vi "observacao.vi"() -> ()   [LabVIEW 2018, in "Shared_160.lvlib"]
uses:
  Shared_160.lvlib
  Control 1.ctl
  System.Windows.Forms
  Global_Telescopio.vi
panel:
  out "statusReadTime":u32
  in  "Internal Dew Point":dbl
  in  "Dew Point 2":dbl
  in  "Humidity 2":dbl
  in  "Wind Speed 2":dbl
  in  "LEAF 2":i32
  in  "ExternalTracking":bool caption="non-sideral"
  out "externalNST":bool
  in  "VARIABLE \nTRACKING":bool
  out "LED VAR TRACKING":bool
  out "LED GUIDER":bool
  out "Led Chave Dome":bool
  out "LED MOUNT":bool
  in  "GUIDER":bool
  in  "DOME":bool
  in  "MOUNT":bool
  out "Weather rec. time":timestamp
  in  "Default":string="DEFAULT"
  out "angCup":string caption="DOME Pos"
  out "TargetCup":string caption="DOME Tar"
  out "domeRisc":bool
  out "element":string
  out "size(s)":i32
  out "timeStatShutterAlert":i32
  out "sendCommandShutter":bool
  out "shutterTimeOld":i32
  out "LEAF":i32
  out "Flag ativo DEC":bool
  out "Flag ativo AH":bool
  out "Flag de erro p/ apagar lampada":bool
  in  "erro lig":i32=3
  in  "erro des":i32=3
  in  "xxz":string
  out "Flag desligar":bool
  out "Flag ligar":bool
  out "Flag Stop":bool
  in  "AUX LAMPADA":bool
  out "Apontou":bool caption="Working Area"
  in  "AUX ABA":bool
  in  "error in (no error)":errorcluster
  out "AH_Destino":dbl format="%.9g"
  out "CONT DEC UTILS":i32
  out "CR DEC UTILS":i32
  out "CONT AH UTILS":i32
  out "CR AH UTILS":i32
  out "Erro PROTEC":i32=5
  out "Erro Lim":i32=5
  out "Flag Alarm":bool
  out "alarm Time":timestamp
  in  "LedPointing":bool=TRUE
  in  "Case Ct":bool=TRUE
  in  "Case Constant\n(See Context Help) 12":bool=TRUE
  in  "Case Constant\n(See Context Help) 11":bool
  in  "Case Constant\n(See Context Help) 8":bool=TRUE
  in  "Case Constant\n(See Context Help) 7":bool=TRUE
  in  "Case Constant\n(See Context Help) 6":bool
  in  "Case Constant\n(See Context Help) 5":bool
  in  "TRUE=HORA\nFALSE=GRAU":bool=TRUE
  in  "Case Constant\n(See Context Help) 4":bool
  in  "Case Constant\n(See Context Help) 3":bool
  in  "Case Constant\n(See Context Help) 2":bool
  in  "Case Constant\n(See Context Help)":bool
  out "TA3":u32
  out "TA2":u32
  out "TF2":u32
  out "TF1":u32
  out "TA1":u32
  out "Tick Cupula":u32
  out "T2 3":u32
  in  "ESTADO ABRIR":string
  in  "ESTADO FECHAR":string
  out "T2 2":u32
  out "T1 2":u32
  out "T2":u32
  out "T1":u32
  out "DEC":string="00 00 00,00"
  out "Hour Angle 2":string="00 00 0,00" caption="AH"
  in  "TIMER TICK":u32
  in  "STOP":bool
  in  "News":bool
  out "AtmosferaStr":string
  in  "BtShutterClose":bool caption="DOME SHUTTER"
  out "HA obs":dbl
  out "Time to Limit":string
  in  "Clear All Messages":bool
  out "FiltroDuplo":bool
  out "ObjCentrado":bool
  out "Timeout PROT":u32
  out "LIMITE":bool
  in  "DestCUP":i16
  in  "DestAH":dbl
  in  "DestDEC":dbl
  in  "M_CUP":i32
  out "TimeoutCUP 2":u32
  out "TimeoutAH 2":u32
  out "TimeoutDEC 2":u32
  out "error out":errorcluster
  out "TUBO_STAT":string
  out "CUP_STAT":string
  out "DEC_STAT":string
  out "AH_STAT":string
  out "FOCO_ENC":string
  out "DEC_ENC":string
  out "AH_ENC":string
  out "RA on Target":bool
  in  "BtOnTatget":bool
  out "Offset DEC":dbl format="%#.2f"
  out "Offset RA":dbl format="%#.2f"
  out "Mount Fine Movement":bool
  out "Mount Gross Movement":bool
  out "subarray":string[][](array[string])
  in  "sair":bool
  out "Saida Path string":string
  out "AUX EDITA RA":string caption="Name"
  out "Sideral time":string caption="ST"
  out "UT":string
  out "FLAG SET COORD":bool
  out "AUX EDITA PMDEC":string caption="Name"
  out "AUX EDITA PMRA":string caption="Name"
  out "AUX EDITA EPOCH":string caption="Name"
  out "AUX EDITA DEC":string caption="Name"
  out "AUX EDITA Name":string caption="Name"
  out "Hour Angle":string="00 00 0,00"
  in  "DECTARGET":string
  in  "AHTARGET":string
  out "Zenital angle":dbl
  out "SlideEnviromental":dbl(slide) caption="Progress ..." scale=0.0..100.0
  out "RA AUX":string
  out "EPOCH AUX":string
  out "SYSTEM MESSAGES":string
  out "Data Acquisition Activity":bool
  out "Auto guider Activity":bool
  out "Security Zone":bool
  out "Precess Data out-of-date":bool
  out "Weather data received":bool
  out "Plataform":bool
  out "B...":bool
  out "Shutter opened":bool
  out "DEC on Target":bool
  out "Dome on Target":bool
  out "Remote User in Control":bool
  out "Air Mass":dbl
  out "Epoch":dbl
  out "Right Ascention":string="00 00 00,00"
  out "Declination":string="00 00 00,00"
  out "Azimuth":dbl
  out "Wind Chill":dbl
  out "Boolean 11":bool
  out "Wind Dir":string
  in  "Int/Ext":bool=TRUE
  out "Temperature":dbl
  out "Humidity":dbl
  out "Dew Point":dbl
  out "Wind Speed":dbl
  out "Pressure":dbl
  out "NAME":string
  out "DEC":string
  out "RA":string
  in  "Tab Control":T1(tab)=enum."Test Only"
  in  "PictureBox":refnum<k24>(container)
  out "pressão atm":string
  out "hum local":string
  out "Temp amb":string
  out "C. AH":i32
  out "DOMO_ENC":string
  out "Proteção":bool
  in  "M_PROT":i32
  out "dt":u32
  out "TUBO":bool[](array[boolean])
  out "CUP":bool[](array[boolean])
  out "DEC":bool[](array[boolean])
  out "RA":bool[](array[boolean])
  in  "statCUP":i32
  in  "statAH":i32
  in  "statDEC":i32
  out "statCUP 2":i32
  out "TimeoutCUP":u32
  out "Azimute cup":u16
  out "PosCUP":i16
  out "dtAUX2":u32
  out "dtAUX3":u32
  out "PosAH":dbl
  out "PosDEC":dbl
  out "dec=":bool
  out "ah=":bool
  in  "CR AH":i32
  in  "CR DEC":i32
  out "C. DEC":i32
  in  "M_AH":i32
  in  "M_DEC":i32
  out "cmdT":string
  in  "Stop All":bool
  in  "Setup, Pointing & Guiding":T2(tab)=enum."POINTING"
  in  "RA Max 2":i32 min=-6 max=23
  in  "RA Min 2":i32 min=-6 max=23
  out "Erro":bool
  in  "MAG Max":dbl min=-9.0 max=100.0
  in  "MAG Min":dbl min=-9.0 max=25.0
  in  "DEC Max":i32 min=-90 max=90
  in  "DEC Min":i32 min=-90 max=90
  in  "RA Max":i32 caption="AH Max" min=-6 max=23
  in  "RA Min":i32 caption="AH Min" min=-6 max=23
  in  "Filter RA":bool
  in  "Slide old":i32
  out "Tot Linhas":i32
  in  "Open BSC":bool
  in  "Slide":dbl(slide) min=0.0 max=24.0 step=0.024 scale format="%#_3g"
  in  "EDIT":bool
  in  "Insert":bool
  out "List File":string
  in  "Upload":bool
  in  "Open":bool
  in  "Save AS":bool
  in  "Save":bool
  in  "Clear ALL":bool
  in  "SET coord":bool
  in  "Delete":bool
  in  "Multicolumn Listbox":i32[](listbox)
  out "ScaleMin":string
  out "ScaleMax":string
  out "DEC obs":dbl format="%.9f"
  out "RA obs":dbl format="%.9f"
  in  "ChkPointPrecessed":bool
  in  "Processa Centragem":bool
  out "PM_DEC":string
  out "PM_RA":string
  out "LedPointing":bool caption="Telescope Pointing"
  out "TimeoutAH":u32
  out "TimeoutDEC":u32
  out "AtualDEC":dbl format="%.9f"
  out "MeanDEC":string
  out "MeanRA":string
  in  "MAG":string
  out "Zenital Angle":string
  out "Air Mass":string
  out "Tempo Obs":string
  in  "BtPointPrecess":bool
  in  "ChkCalGlobal":bool=TRUE
  in  "ChkCalLocal":bool caption="Use Local Zero"
  in  "ChkPoinLampOFF":bool=TRUE
  in  "ChkPointRNA":bool
  in  "ChkModel":bool=TRUE
  in  "ChkWindDown":bool
  in  "ChkOpenShutter":bool
  in  "ChkDomeEnable":bool
  out "LedPointWorkArea":bool caption="Working Area"
  in  "BtTargetPoint":bool
  out "StrPointTargetDEC":string caption="Declination"
  out "StrPointTargetRA":string caption="Right Ascension"
  in  "BtPointObjClear":bool
  in  "StrPointObjPMDEC":string caption="DEC Proper Motion"
  in  "StrPointObjPMRA":string caption="RA Proper Motion"
  in  "StrPointObjName":string caption="Name"
  in  "StrPointObjEpoch":string caption="Epoch"
  in  "StrPointObjDEC":string caption="Declination"
  in  "StrPointObjRA":string caption="Right Ascension"
  out "MOV_IDX_DEC":bool
  out "MOV_IDX_AH":bool
  out "LatchDeslocDEC":dbl caption="DEC"
  out "LatchDeslocRA":dbl caption="RA"
  in  "ClearDeslocDEC":bool
  in  "ClearDeslocRA":bool
  out "DeslocDEC":dbl caption="DEC" format="%#.1f"
  out "DeslocRA":dbl caption="RA" format="%#.1f"
  in  "Delete Calagem":bool
  in  "Global":bool caption="Local"
  in  "Calagem":bool
  in  "Up HS":bool
  in  "Right HS":bool
  in  "Down HS":bool
  in  "Left HS":bool
  in  "Velocity (arcsec/sec)":i32(slide) min=0 max=600 scale=0.0..600.0
  in  "BtPrecGO":bool
  in  "BtPrecCentrar":bool
  in  "PreciseOffsetDEC":dbl caption="DEC" min=-10000.0 max=10000.0 step=1.0 format="%.3g"
  in  "PreciseOffsetRA":dbl caption="RA . cos(delta)" min=-10000.0 max=10000.0 step=1.0 format="%.3g"
  in  "Habilita Movimento":bool=TRUE
  in  "Y STAR":i32=1 min=1 max=400 step=1
  in  "X STAR":i32=1 min=1 max=400 step=1
  in  "XY CENTER":bool
  in  "Y CENTER":i32=1 min=1 max=400 step=1
  in  "X CENTER":i32=1 min=1 max=400 step=1
  in  "ClearRA":bool
  in  "ClearDEC":bool
  in  "DEC RATE":i32 min=-2000 max=2000 step=1
  in  "RA  RATE":i32 min=-2000 max=2000 step=1
  in  "focusStop":bool
  in  "Velocity":dbl(slide)=1.0 caption="(max = 500 u/s)" min=0.1 max=100.0 step=1.0 scale=0.1..100.0
  in  "focusHome":bool
  out "focusStatus":string="            Focus Status"
  out "focuAlarm":bool caption="Motor temp."
  out "focusHoming":bool caption="Homing"
  out "focusMoving":bool caption="Moving"
  out "focusConnected":bool
  out "focusInitialized":bool
  in  "SetDefaultFocus":bool
  out "Foco":dbl(slide) caption="1" scale=0.0..50000.0
  in  "Setpoint":dbl=200.0 caption="Target" min=0.0 max=50700.0 step=1.0
  in  "focusGo":bool
  in  "Focus +":bool caption="Focus Out (+)"
  in  "Focus -":bool caption="Focus In (-)"
  in  "New Angle":string="    0.0"
  out "Default Angle":string="      0.00"
  in  "SetRotatorDefAngle":bool
  in  "Set Rotator Angle":bool
  out "Rotator Angle":string="  0.00" caption="for  GUIDING"
  in  "OpenShutterPassword":string caption="Senha para Abrir"
  in  "BtShutterClose":bool
  in  "BtShutterOpen":bool
  out "trapeiraAberta":bool caption="Open"
  out "trapeiraMovendo":bool caption="Moving"
  out "trapeiraFechada":bool caption="Closed"
  out "Command":string
  in  "CCW":bool
  in  "BtParavStop":bool
  in  "BtParavUp":bool
  in  "BtParavDown":bool
  out "StatDome":string caption="Control State"
  in  "BtDomeSTOP":bool
  in  "BtDomeGO":bool caption="DOME"
  in  "DomeNewPos":i32=30 caption="New Position" min=1 max=360
  out "AngCup":i16 caption="Position"
  in  "CW":bool
  in  "BtUtilPark":bool
  out "LED ACTION":bool
  out "LED MODE":bool
  in  "ACTION":bool
  in  "MODE":bool
  in  "PROTEÇÃO":bool
  in  "STOP":bool
  in  "Enable Centragem":bool=TRUE
  in  "GO":bool
  in  "StrPointObjDEC 2":string caption="DEC"
  in  "StrPointObjRA 2":string caption="AH"
  out "MOVING":bool
  in  "FLAT-FIELD":bool
  in  "ECASS":bool
  in  "BtUtilZenith":bool
  in  "TabInstrumento":T3(tab)=enum."Cam 1"
  out "Posição Rede":i32=10 caption="Largura da Fenda" min=10 max=5000 step=1
  in  "HomePrisma":T4 caption="DOME"
  in  "HomeEspelho":T4 caption="DOME"
  in  "HomeFenda":T4 caption="DOME"
  in  "IronArc":bool=TRUE
  out "Boolean":bool
  out "Largura da Fenda 2":dbl=10.0 caption="Largura da Fenda" min=10.0 max=5000.0 step=1.0
  in  "Prisma das Lâmpadas":bool
  out "Position":string
  in  "Largura da Fenda":dbl=10.0 min=10.0 max=5000.0 step=1.0
  in  "Go Largura da Fenda":bool caption="DOME"
  in  "Angulo da rede de difração":i32=10 caption="Ângulo da Rede" min=10 max=99989 step=1
  in  "Go Angulo de Difração":bool caption="DOME"
  in  "Incand":bool=TRUE
  in  "Neon":bool=TRUE
  in  "Cathode":bool=TRUE
  out "Ang. Fenda":dbl
  in  "Go_Coudé":bool
  in  "Radio Buttons":enum32{"Azul", "Visível", "Vermelho"}(radio)
  out "EndTime":u32
  out "ledAzul":bool
  out "ledVisivel":bool
  out "ledVermelho":bool
  in  "MENSAGEM":string="EM MOVIMENTO"
  out "MENSAGEM 2":string="EM MOVIMENTO"
  out "#2":bool
  out "#3":bool
  out "#4":bool
  out "PosSecundario":bool
  out "Cjto_3":bool
  out "EspAtual":string
  out "parou":bool
  out "parou 2":bool
  out "Posição Espelho":dbl=10.0 caption="Largura da Fenda" min=10.0 max=5000.0 step=1.0
  out "parou 3":bool
  out "Output Message":string
  in  "stopEcass":bool
  out "SlideEcass":u8(slide) caption="Espelho movendo..." max=100 scale=0.0..100.0
  out "LedRep":bool
  out "LedCal":bool
  in  "Sent_EspLampCass":bool
  out "LedHe":bool
  out "LedNe":bool
  in  "He-Ar":bool
  in  "Ne":bool
  in  "Mensage Alarme":string="To light up close the Shutter !"
  out "CoudeSel":bool
  in  "Coude":bool
  in  "BtCalFlatField":bool
  in  "ChkCalLamp4":bool
  in  "ChkCalLamp3":bool
  in  "ChkCalLamp2":bool
  in  "ChkCalLamp1":bool
  in  "BtCalTurnOff":bool
  in  "BtCalTurnOn":bool
  out "StrongSel":bool
  out "MediumSel":bool
  out "WeakSel":bool
  in  "Strong":bool
  in  "Medium":bool
  in  "Weak":bool
  # "TELESCOPE CONTROL SYSTEM\nPICO DOS DIAS OBSERVATORY"
  # "Status Information"
  # "System Positions"
  # "Environmental Status"
  # "(+/-2)"
  # "mBar"
  # "INT"
  # "EXT"
  # "o"
  # "C"
  # "Km/h"
  # "%"
  # "o"
  # "C"
  # "o"
  # "C"
  # "CLOUSURE LIMITS"
  # "Wind Speed            >  70 Km/h\nRelative Humidity    >  97 %\nInternal Dewpoint  <  0.5  C\nExternal Dewpoint <  1.0  C"
  # "OBJECT"
  # "TRACKING ENABLE"
  # "Conector 4"
  # "Conector 3"
  # "ALARME\nATENÇÃO\nERROS\nOCUPADO"
  # "Proteção\n\nTracking\nVar_Track"
  # "PLATAF\nLCB\nTRAP\nPARAV"
  # "Rapido\nLigeiro\nFino\nRun"
  # "Rapido\nCW\nCCW\nMoving"
  # "Motor\nIDX_Rdy\nManual"
  # "TRAP_RUN\nTRAP_FCH\nTRAP_ABT"
  # "BSC FILTERS"
  # "LIST FILE"
  # "OBJECT INPUT"
  # "TARGET"
  # "OPTIONS"
  # "MANUAL OFFSET"
  # "PRECISE OFFSET"
  # "N"
  # "E"
  # "W"
  # "arcsec"
  # "arcsec"
  # "S"
  # "DISPLACEMENT"
  # "CALAGEM"
  # "PODE NÃO FUNCIONAR CORRETAMENTE!"
  # "STAR CENTERING"
  # "AUTO-GUIDER COORDINATES"
  # "INTERNAL VAR. TRACKING"
  # "1) Entrar X e Y do cursor do Autoguider correspondente à posição de centragem nas entradas X CENTER e Y CENTER. \n2) Após apontamento, entrar em X STAR e Y STAR os valores de X e Y do Autoguider com o \"Guide Box\" sobre o objeto apontado. \n3) Clicar em MOVE STAR TO CENTER."
  # "(instrument)"
  # "May take many\ntens of seconds"
  # "Continuous Movement"
  # "%"
  # "ATENÇÃO:\nO Rotator ainda não está integrado ao sistema de controle e como sua posição afeta a guiagem, sempre que o rotator for girado manualmente é necessário digitar o valor de sua nova posição no controle \"New Angle\" e pressionar \"SET NEW\".\n\nPressionar \"SET NEW\" ou \"SET DEFAULT\" não gira o rotator!"
  # "ROTATION"
  # "WINDSCREEN"
  # "SHUTTER"
  # "Covers"
  # "FIXED POSITIONS"
  # "Acquisition System\nON TARGET command"
  # "Select one Mirrror"
  # "Mirror #2"
  # "Mirror #3"
  # "Mirrors Drivers"
  # "Lâmpadas de Calibração"
  # "Espelho das Lâmpadas de Calibração"
  # "Posição"
  # "Repouso"
  # "Ativo"
  # "LIGA"
  # "LIGA"
  # "DESL."
  # "DESL."
  # "Espelho do Eucalyptus"
  # "Roda de filtros"
  # "Posição"
  # "Repouso"
  # "Ativo"
  # "Espelho de Campo"
  # "Recuar"
  # "Avançar"
  # "Rápido"
  # "Lento"
  # "CALIBRATION LAMPS"
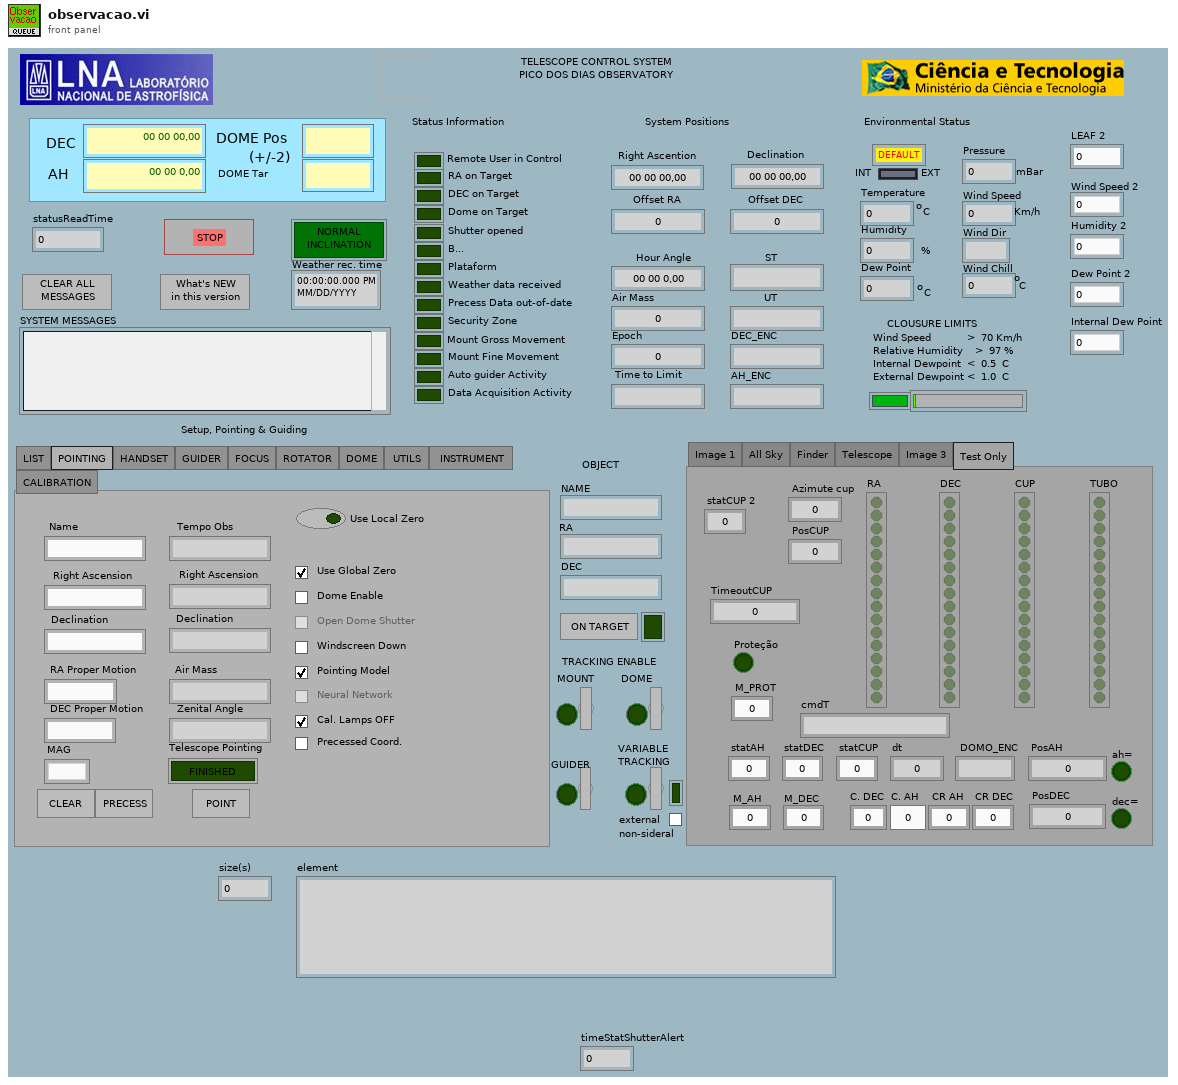
[diagram p1: front panel]
types:
  T1 = enum32{"Image 1", "All Sky", "Finder", "Telescope", "Image 3", "Test Only"}
  T2 = enum32{"LIST", "POINTING", "HANDSET", "GUIDER", "FOCUS", "ROTATOR", "DOME", "UTILS ", " INSTRUMENT ", "CALIBRATION"}
  T3 = enum32{"Coude", "Casseg.", "Eucalyp.", "Cam 1", "Cam 2", "Cam IV.", "Polarim.", "Fotrap"}
  T4 = typedef "Control 1.ctl" = bool
  T5 = enum8{"Enabled", "Disabled", "Disabled and Grayed Out"}
  T6 = enum32{"Page Enabled", "Page Disabled", "Page Disabled & Grayed"}
  T7 = enum16{"open", "replace", "create", "open or create", "replace or create", "replace or create with confirmation"}
  T8 = enum16{"open", "open or create", "create or replace", "create"}
  T9 = enum16{"open", "open or create", "create or replace", "create", "open (read only)"}
  T10 = typedef "LVRemotePanelConnectionsTypeDef.ctl" = cluster{"VI Name":string, "Remote":string, "UserName":string, "Port":i32, "Status":enum32{"Viewing", "Waiting For Control", "Controlling"}, "Create Time":timestamp, "Status Time":timestamp, "Control End Time":timestamp}[]
  T11 = cluster{"absolute":bool, "alarm":bool, "broker":string, "cmd":cluster{"clientId":dbl, "clientTransactionId":dbl, "clientName":string, "action":string}, "connected":bool, "controller":string, "device":string, "error":string, "homing":bool, "initialized":bool, "isMoving":bool, "maxSpeed":dbl, "maxStep":dbl, "position":dbl, "tempComp":bool, "tempCompAvailable":bool, "temperature":dbl, "timestamp":string, "version":string}
  T12 = cluster{"clientId":dbl, "clientTransactionId":dbl, "clientName":string, "action":string}
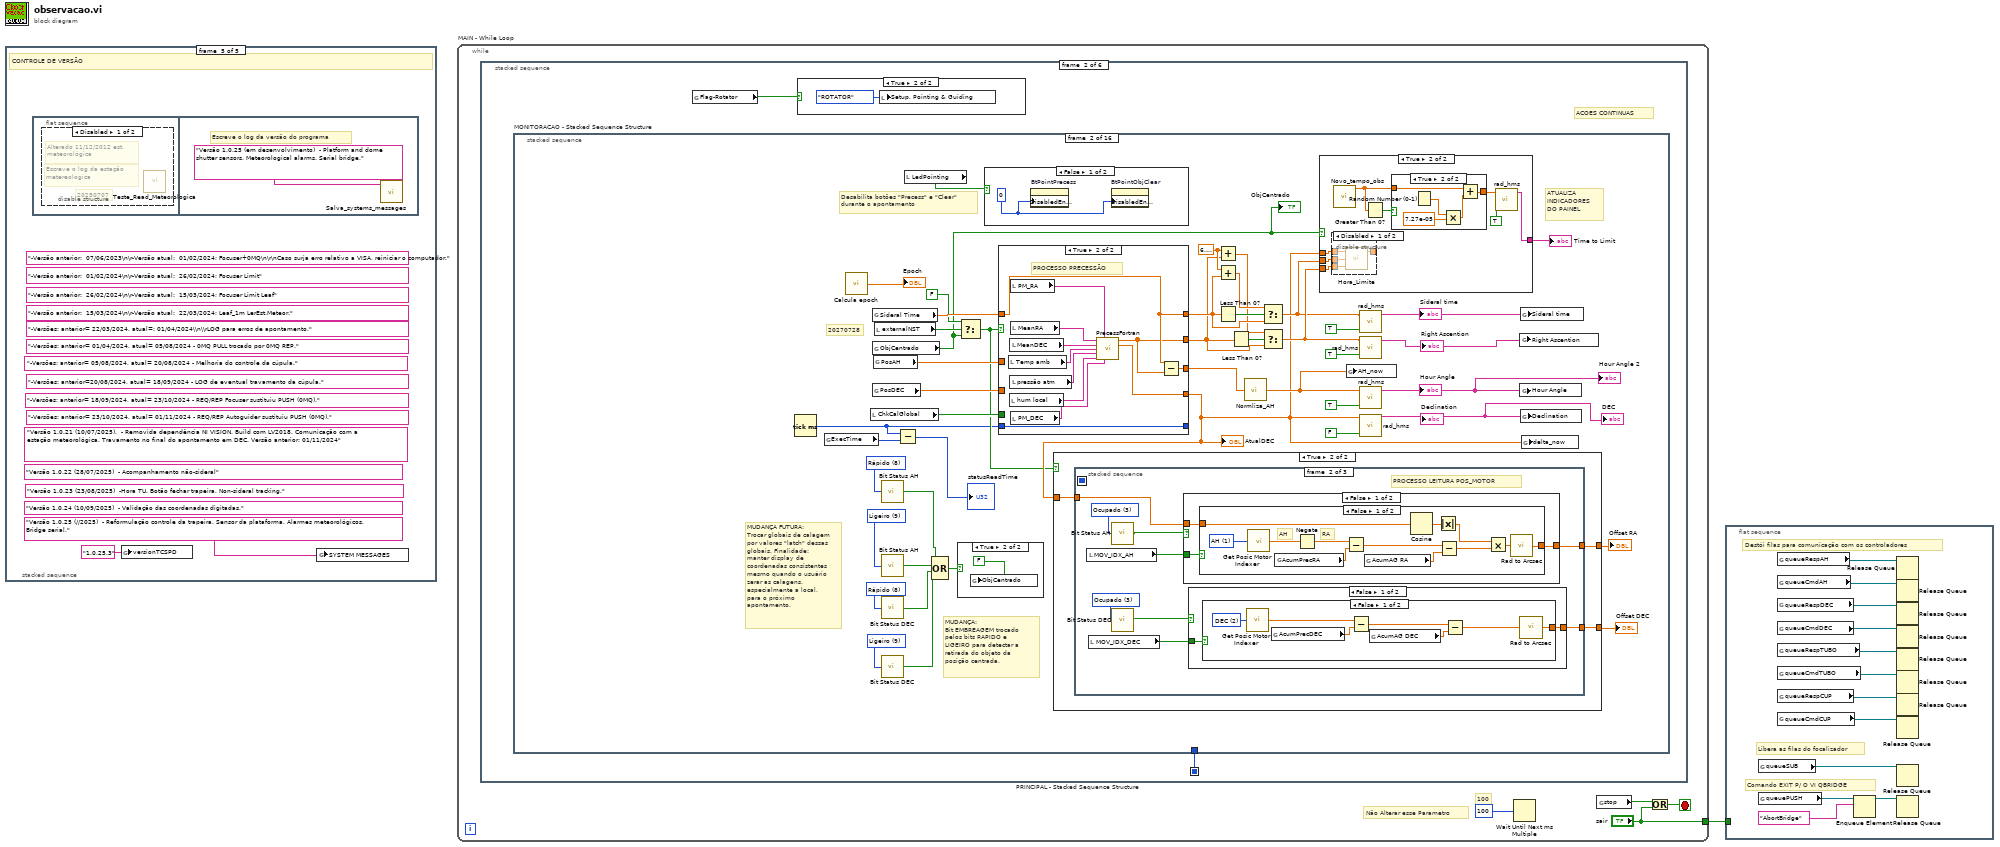
[diagram p0: block diagram]
diagram:
  n1 = stacked-sequence {
    frame #0 {
      w3 = ""
      w5 = 0 ("estado")
      w4 = ""
      w6 = TRUE ("ChkDomeEnable")
      w2 = FALSE ("Set aux")
      # "RESET DE VARIÁVEIS E CONTROLES"
      n2 = local write "FLAG SET COORD"(w2) -> ()
      n3 = local write "DEC on Target"(w2) -> ()
      n4 = local write "Dome on Target"(w2) -> ()
      n5 = local write "MOUNT"(w2) -> ()
      n6 = local write "ACTION"(w2) -> ()
      n7 = local write "GO"(w2) -> ()
      n8 = local write "MOV_IDX_AH"(w2) -> ()
      n9 = local write "MOV_IDX_DEC"(w2) -> ()
      n10 = local write "Flag ativo AH"(w2) -> ()
      n11 = local write "MOVING"(w2) -> ()
      n12 = local write "Flag ativo DEC"(w2) -> ()
      n13 = local write "RA on Target"(w2) -> ()
      n14 = local write "Erro"(w2) -> ()
      n15 = local write "ChkPointPrecessed"(w2) -> ()
      n16 = local write "ChkOpenShutter"(w2) -> ()
      n17 = local write "Enable Centragem"(w2) -> ()
      n18 = local write "Cathode"(w2) -> ()
      n19 = local write "Neon"(w2) -> ()
      n20 = local write "Incand"(w2) -> ()
      n21 = local write "Apontou"(w2) -> ()
      n22 = local write "Precess Data out-of-date"(w2) -> ()
      n23 = local write "Flag Stop"(w2) -> ()
      n24 = local write "MODE"(w2) -> ()
      n25 = local write "LED ACTION"(w2) -> ()
      n26 = local write "LED MODE"(w2) -> ()
      n27 = local write "Flag de erro p/ apagar lampada"(w2) -> ()
      n28 = local write "ExternalTracking"(w2) -> ()
      n29 = local write "externalNST"(w2) -> ()
      n30 = local write "trapeiraFechada"(w2) -> ()
      n31 = local write "trapeiraMovendo"(w2) -> ()
      n32 = local write "trapeiraAberta"(w2) -> ()
      n33 = global write "Global_Telescopio.vi" "Default Met"(w2) -> ()
      n34 = global write "Global_Telescopio.vi" "Flag-Rotator"(w2) -> ()
      n35 = global write "Global_Telescopio.vi" "Centragem Via Aquisicao"(w2) -> ()
      n36 = global write "Global_Telescopio.vi" "Botão GO = STOP"(w2) -> ()
      n37 = global write "Global_Telescopio.vi" "AQ Offset Mov"(w2) -> ()
      n38 = global write "Global_Telescopio.vi" "STOP ALL"(w2) -> ()
      n39 = global write "Global_Telescopio.vi" "Bit RX Aquis"(w2) -> ()
      n40 = global write "Global_Telescopio.vi" "Bit RX Guider"(w2) -> ()
      n41 = global write "Global_Telescopio.vi" "Correção Guider"(w2) -> ()
      n42 = global write "Global_Telescopio.vi" "CalGlobal"(w2) -> ()
      n43 = global write "Global_Telescopio.vi" "CalLocal"(w2) -> ()
      n44 = global write "Global_Telescopio.vi" "ObjCentrado"(w2) -> ()
      n45 = global write "Global_Telescopio.vi" "LIMITE"(w2) -> ()
      n46 = global write "Global_Telescopio.vi" "ExtDEC correction"(w2) -> ()
      n47 = global write "Global_Telescopio.vi" "ExtRA correction"(w2) -> ()
      n48 = global write "Global_Telescopio.vi" "ExtDEC_shift"(w3) -> ()
      n49 = global write "Global_Telescopio.vi" "ExtRA_shift"(w3) -> ()
      n50 = local write "TIMER TICK"(w5) -> ()
      n51 = local write "erro lig"(w5) -> ()
      n52 = local write "erro des"(w5) -> ()
      n53 = local write "statDEC"(w5) -> ()
      n54 = local write "statAH"(w5) -> ()
      n55 = local write "statCUP"(w5) -> ()
      n56 = local write "Tick Cupula"(w5) -> ()
      n57 = local write "CR AH"(w5) -> ()
      n58 = local write "CR DEC"(w5) -> ()
      n59 = global write "Global_Telescopio.vi" "CupStartPos"(w5) -> ()
      n60 = local write "StrPointTargetRA"(w4) -> ()
      n61 = local write "StrPointTargetDEC"(w4) -> ()
      n62 = local write "AUX EDITA RA"(w4) -> ()
      n63 = local write "AUX EDITA EPOCH"(w4) -> ()
      n64 = local write "AUX EDITA PMRA"(w4) -> ()
      n65 = local write "Tempo Obs"(w4) -> ()
      n66 = local write "RA"(w4) -> ()
      n67 = local write "DEC"(w4) -> ()
      n68 = local write "NAME"(w4) -> ()
      n69 = local write "MAG"(w4) -> ()
      n70 = local write "StrPointObjName"(w4) -> ()
      n71 = local write "StrPointObjRA"(w4) -> ()
      n72 = local write "StrPointObjDEC"(w4) -> ()
      n73 = local write "StrPointObjEpoch"(w4) -> ()
      n74 = local write "StrPointObjPMRA"(w4) -> ()
      n75 = local write "StrPointObjPMDEC"(w4) -> ()
      n76 = local write "AUX EDITA Name"(w4) -> ()
      n77 = local write "AUX EDITA DEC"(w4) -> ()
      n78 = local write "AUX EDITA PMDEC"(w4) -> ()
      n79 = local write "ScaleMin"(w4) -> ()
      n80 = local write "Zenital Angle"(w4) -> ()
      n81 = local write "Air Mass"(w4) -> ()
      n82 = local write "Position"(w4) -> ()
      n83 = local write "angCup"(w4) -> ()
      n84 = local write "Position"(w4) -> ()
      n85 = local write "angCup"(w4) -> ()
      n86 = local write "ScaleMax"(w4) -> ()
      n87 = local write "ChkDomeEnable"(w6) -> ()
      n88 = local write "AUX ABA"(w6) -> ()
      n89 = local write "AUX LAMPADA"(w6) -> ()
    }
    frame #1 {
      w8 = "C:\\TCS\\SETUP\\METEOR_DEFAULT.DAT"
      w11 = TRUE ("GUIDING")
      w14 = string[][] [] ("Item Names")
      w16 = T5."Enabled" ("Disabled")
      # "TU safe"
      # "INICIALIZAÇÃO DE PROPRIEDADES"
      n90 = property on="Setup, Pointing & Guiding" class="TabCtl (strict)"() -> ("Pages"=w13:refnum<vi>[])  [unwired: 2 in, 2 out]
      n91 = for {
        tunnel: w13 -> [w32] mode=indexing
        # "HABILITA TODAS AS ABAS"
        n92 = property class="Page"(reference=w32, "Page Enabled State"=T6."Page Enabled") -> ()  [unwired: 1 in, 2 out]
      }
      n93 = property on="Setup, Pointing & Guiding" class="TabCtl (strict)"("Page Selector Visible"=TRUE) -> ()  [unwired: 2 in, 2 out]
      n94 = property on="BtPointObjClear" class="Bool"("DisabledEnum"=w16) -> ()  [unwired: 2 in, 2 out]
      n95 = property on="BtPointPrecess" class="Bool"("DisabledEnum"=w16) -> ()  [unwired: 2 in, 2 out]
      n96 = property on="PROTEÇÃO" class="Bool (strict)"("Disabled"=w16) -> ()  [unwired: 2 in, 2 out]
      n97 = property on="FLAT-FIELD" class="Bool (strict)"("Disabled"=w16) -> ()  [unwired: 2 in, 2 out]
      n98 = property on="BtUtilZenith" class="Bool (strict)"("Disabled"=w16) -> ()  [unwired: 2 in, 2 out]
      n99 = property on="ECASS" class="Bool (strict)"("Disabled"=w16) -> ()  [unwired: 2 in, 2 out]
      n100 = property on="BtUtilPark" class="Bool (strict)"("Disabled"=w16) -> ()  [unwired: 2 in, 2 out]
      n101 = property on="ACTION" class="Bool (strict)"("Disabled"=T5."Disabled and Grayed Out") -> ()  [unwired: 2 in, 2 out]
      n102 = property on="Setup, Pointing & Guiding" class="TabCtl (strict)"("MultColors"=TRUE ("Allow Multiple Colors")) -> ()  [unwired: 2 in, 2 out]
      n103 = property on="LedPointWorkArea" class="Bool (strict)"("Visible"=TRUE ("GUIDING")) -> ()  [unwired: 2 in, 2 out]
      n104 = property on="Mensage Alarme" class="Str"("Visible"=FALSE, "Blinking"=TRUE) -> ()  [unwired: 2 in, 2 out]
      n105 = property on="LedPointing" class="Bool (strict)"("Visible"=FALSE ("Set aux")) -> ()  [unwired: 2 in, 2 out]
      n106 = String To Path(string=w8) -> (path=w10:path)
      n107 = call <vilib>:"Check if File or Folder Exists.vi"("path"=w10) -> ("file or folder exists?"=w9:bool)  [unwired: 8 in, 2 out]
      n108 = case shown="False" w9 {
        tunnel: w8 -> [w27 _]
        frame False {
          n109 = global read "Global_Telescopio.vi" "weatherCfgDef"() -> (w30:string[])
          n110 = Build Array(w30) -> (w29:string[][])
          n111 = Transpose 2D Array(2D array=w29) -> (transposed array=w28:string[][])
          n112 = call "salvaexel.vi"("appended array"=w28, "file name p/ exell"=w27) -> ()  [unwired: 1 in, 1 out]
        }
        frame True {
        }
      }
      n113 = call "Get host time.vi"() -> ("BR current time"=w7:timestamp)  [unwired: 8 in, 3 out]
      n114 = control-ref of="BtTargetPoint"() -> (w19:refnum<vi>)
      n115 = control-ref of="Erro"() -> (w21:refnum<vi>)
      n116 = property on="domeRisc" class="Bool"("Visible"=FALSE ("Set aux")) -> ()  [unwired: 2 in, 2 out]
      n117 = property on="domeRisc" class="Bool"("Blinking"=w11) -> ()  [unwired: 2 in, 2 out]
      n118 = global write "Global_Telescopio.vi" "weather160 PUB time"(w7) -> ()
      n119 = global write "Global_Telescopio.vi" "weather 0MQ last time"(w7) -> ()
      n120 = property class="Bool (strict)"(reference=w21, "Boolean Text.Text"="") -> ()  [unwired: 1 in, 2 out]
      n121 = property class="Bool"(reference=w19, "Boolean Text.Text"="POINT") -> ()  [unwired: 1 in, 2 out]
      n122 = property on="Multicolumn Listbox" class="MCListbox (strict)"("Item Names"=w14) -> ()  [unwired: 2 in, 2 out]
      n123 = local write "subarray"(w14) -> ()
      "domeRisc" <- w11
    }
    frame #2 {
      w35 = "REPOUSO" ("y")
      # "20250927 Cria filas para comunicação com Bridge serial.vi"
      # "TU safe"
      # "MUDANÇA 22/6/11:\nÂngulo do rotator muda ao reiniciar o PC."
      # "Iinicializando o timer do shutter"
      # "INICIALIZAÇÃO DE CONTROLES E FILAS DE COMUNICAÇÃO"
      n124 = stacked-sequence {
        frame #0 {
          n125 = Obtain Queue(name (unnamed)="queueCmdAH", element data type="") -> (queue out=w48:refnum<queue>)  [unwired: 3 in, 2 out]
          n126 = global write "Global_Telescopio.vi" "queueCmdAH"(w48) -> ()
          n127 = Obtain Queue(name (unnamed)="queueRespAH", element data type="") -> (queue out=w45:refnum<queue>)  [unwired: 3 in, 2 out]
          n128 = global write "Global_Telescopio.vi" "queueRespAH"(w45) -> ()
        }
        frame #1 {
          n129 = Obtain Queue(name (unnamed)="queueCmdDEC", element data type="") -> (queue out=w54:refnum<queue>)  [unwired: 3 in, 2 out]
          n130 = global write "Global_Telescopio.vi" "queueCmdDEC"(w54) -> ()
          n131 = Obtain Queue(name (unnamed)="queueRespDEC", element data type="") -> (queue out=w51:refnum<queue>)  [unwired: 3 in, 2 out]
          n132 = global write "Global_Telescopio.vi" "queueRespDEC"(w51) -> ()
        }
        frame #2 {
          n133 = Obtain Queue(name (unnamed)="queueCmdTUBO", element data type="") -> (queue out=w60:refnum<queue>)  [unwired: 3 in, 2 out]
          n134 = global write "Global_Telescopio.vi" "queueCmdTUBO"(w60) -> ()
          n135 = Obtain Queue(name (unnamed)="queueRespTUBO", element data type="") -> (queue out=w57:refnum<queue>)  [unwired: 3 in, 2 out]
          n136 = global write "Global_Telescopio.vi" "queueRespTUBO"(w57) -> ()
        }
        frame #3 {
          n137 = Obtain Queue(name (unnamed)="queueCmdCUP", element data type="") -> (queue out=w66:refnum<queue>)  [unwired: 3 in, 2 out]
          n138 = global write "Global_Telescopio.vi" "queueCmdCUP"(w66) -> ()
          n139 = Obtain Queue(name (unnamed)="queueRespCUP", element data type="") -> (queue out=w63:refnum<queue>)  [unwired: 3 in, 2 out]
          n140 = global write "Global_Telescopio.vi" "queueRespCUP"(w63) -> ()
        }
      }
      n141 = call "Get host time.vi"() -> ("BR current time"=→"alarm Time":timestamp)  [unwired: 8 in, 3 out]
      n142 = global read "Global_Telescopio.vi" "rotator_def"() -> (w34:string)
      n143 = global read "Global_Telescopio.vi" "Instrum"() -> (w39:u16)
      n144 = local write "Multicolumn Listbox"(i32[] [0] ("Multicolumn Listbox")) -> ()
      n145 = local write "ESTADO FECHAR"(w35) -> ()
      n146 = local write "TabInstrumento"(w39) -> ()
      n147 = property on="TabInstrumento" class="TabCtl (strict)"("Disabled"=u8 0) -> ()  [unwired: 2 in, 2 out]
      n148 = local write "ESTADO ABRIR"(w35) -> ()
      n149 = local write "Rotator Angle"(w34) -> ()
      n150 = local write "Default Angle"(w34) -> ()
      n151 = global write "Global_Telescopio.vi" "guide_ang"(w34) -> ()
      n152 = local write "StatDome"("Stopped" ("Status")) -> ()
      n153 = local write "xxz"("inicio") -> ()
      "Flag Alarm" <- FALSE ("Visible")
      "shutterTimeOld" <- 0 ("shutterTimeOld")
      "sendCommandShutter" <- FALSE ("writeShutterLog")
      "timeStatShutterAlert" <- 0 ("timeStatShutterAlert")
    }
    frame #3 {
      w69 = u8 0 ("Disabled")
      w70 = "OFF"
      w74 = "focusQueue" ("string")
      w75 = ""
      w84 = u16 4 items=["ZERO", "AH", "DEC", "TUBO", "CUP"] ("Controlador")
      w83 = u16 3 items=["ZERO", "AH", "DEC", "TUBO", "CUP"] ("Controlador")
      w81 = u16 2 items=["ZERO", "AH", "DEC", "TUBO", "CUP"] ("Controlador")
      w85 = "PROG" ("Comando")
      w86 = "RESET" ("Comando")
      w80 = u16 1 items=["ZERO", "AH", "DEC", "TUBO", "CUP"] ("Controlador")
      # "Inicializa ClientTransactionId"
      # "Cria as filas de comunicação\ncom 0MQ_Bridge_Foco.vi"
      # "ZeroMQ"
      # "0- Alarme\n1-Atenção\n2-Erro\n3-Ocupado\n******************\n4-Proteção\n5-Embreagem\n6-Tracking\n7-Var.Track\n8-Rápido\n9-Ligeiro\n10-Médio\n11-Lento\n12-Em movimento\n13-TBD\n14-TBF\n15-TBF\n16-TBF"
      # "RESET DOS CONTROLADORES E INICIALIZAÇÃO DAS FILAS DO FOCALIZADOR"
      n154 = call "Monta Comando.vi"("Comando"=w86, "Dispositivo"=w85, "Controlador"=w80) -> ()  [unwired: 2 in, 5 out]
      n155 = property on="Focus +" class="Bool (strict)"("BoolText.Text"=w70) -> ()  [unwired: 2 in, 2 out]
      n156 = property on="Focus -" class="Bool (strict)"("BoolText.Text"=w70) -> ()  [unwired: 2 in, 2 out]
      n157 = Concatenate Strings(w74, "PUSH" ("string")) -> (w77:string)
      n158 = Concatenate Strings(w74, "SUB" ("string")) -> (w76:string)
      n159 = call "Monta Comando.vi"("Comando"=w86, "Dispositivo"=w85, "Controlador"=w81) -> ()  [unwired: 2 in, 5 out]
      n160 = Wait (ms)(milliseconds to wait=u32 2000) -> ()  [unwired: 1 out]
      n161 = global write "Global_Telescopio.vi" "transactionId0MQ"(u64 0 ("transactionId0MQ")) -> ()
      n162 = Obtain Queue(name (unnamed)=w76, element data type=w75) -> (queue out=w73:refnum<queue>)  [unwired: 3 in, 2 out]
      n163 = Obtain Queue(name (unnamed)=w77, element data type=w75) -> (queue out=w72:refnum<queue>)  [unwired: 3 in, 2 out]
      n164 = call "Monta Comando.vi"("Comando"=w86, "Dispositivo"=w85, "Controlador"=w83) -> ()  [unwired: 2 in, 5 out]
      n165 = global write "Global_Telescopio.vi" "queueSUB"(w73) -> ()
      n166 = global write "Global_Telescopio.vi" "queuePUSH"(w72) -> ()
      n167 = call "Monta Comando.vi"("Comando"=w86, "Dispositivo"=w85, "Controlador"=w84) -> ()  [unwired: 2 in, 5 out]
      n168 = property on="Focus -" class="Bool (strict)"("Disabled"=w69) -> ()  [unwired: 2 in, 2 out]
      n169 = property on="Focus +" class="Bool (strict)"("Disabled"=w69) -> ()  [unwired: 2 in, 2 out]
      n170 = property on="Setpoint" class="DigNum (strict)"("Disabled"=w69) -> ()  [unwired: 2 in, 2 out]
    }
    frame #4 {
      (unwired) "Versão 1.0.24 (10/09/2025)  - Validação das coordenadas digitadas." ("message")
      (unwired) "Versão 1.0.23 (23/08/2025)  -Hora TU. Botão fechar trapeira. Non-sideral tracking." ("message")
      (unwired) "Versão 1.0.22 (28/07/2025)  - Acompanhamento não-sideral" ("message")
      (unwired) "-Versões: anterior= 23/10/2024, atual= 01/11/2024 - REQ/REP Autoguider sustituiu PUSH (0MQ)." ("SYSTEM MESSAGES")
      (unwired) "-Versões: anterior= 18/09/2024, atual= 23/10/2024 - REQ/REP Focuser sustituiu PUSH (0MQ)." ("SYSTEM MESSAGES")
      (unwired) "Versão 1.0.21 (10/07/2025).  - Removida dependência NI VISION. Build com LV2018. Comunicação com a estação meteorológica. Travamento no final do apontamento em DEC. Versão anterior: 01/11/2024" ("SYSTEM MESSAGES")
      (unwired) "-Versões: anterior= 05/08/2024, atual= 20/08/2024 - Melhoria do controle da cúpula." ("SYSTEM MESSAGES")
      (unwired) "-Versões: anterior=20/08/2024, atual= 18/09/2024 - LOG de eventual travamento da cúpula." ("SYSTEM MESSAGES")
      (unwired) "-Versões: anterior= 01/04/2024, atual= 05/08/2024 - 0MQ PULL trocado por 0MQ REP." ("SYSTEM MESSAGES")
      (unwired) "-Versões: anterior= 22/03/2024, atual=: 01/04/2024\\n\\rLOG para erros de apontamento." ("SYSTEM MESSAGES")
      (unwired) "-Versão anterior:  26/02/2024\n\r-Versão atual:  15/03/2024; Focuser Limit Leaf" ("SYSTEM MESSAGES")
      (unwired) "-Versão anterior:  01/02/2024\n\r-Versão atual:  26/02/2024; Focuser Limit" ("SYSTEM MESSAGES")
      (unwired) "-Versão anterior:  15/03/2024\n\r-Versão atual:  22/03/2024; Leaf_1m LerEst.Meteor." ("SYSTEM MESSAGES")
      (unwired) "-Versão anterior:  07/06/2023\n\r-Versão atual:  01/02/2024; Focuser+0MQ\n\r\nCaso surja erro relativo a VISA, reiniciar o computador." ("SYSTEM MESSAGES")
      # "CONTROLE DE VERSÃO"
      n171 = flat-sequence {
        frame #0 {
          n172 = disable-structure shown="Disabled" {
            frame Disabled {
              # "20250707"
              # "Escreve o log da estação\nmetereologica"
              # "Alterado 11/12/2012 est.\nmeteorológica"
              n173 = call "Teste_Read_Meteorologica.vi"() -> ()  [unwired: 2 in, 1 out]
            }
            frame Enabled {
            }
          }
        }
        frame #1 {
          # "Escreve o log da versão do programa"
          n174 = call "Salva_systems_messages.vi"("Mensagem"="Versão 1.0.25 (em desenvolvimento)  - Platform and dome shutter sensors. Meteorological alarms. Serial bridge." ("message")) -> ()  [unwired: 5 in]
        }
      }
      n175 = global write "Global_Telescopio.vi" "versionTCSPD"("1.0.25.3" ("versionTCSPD")) -> ()
      n176 = global write "Global_Telescopio.vi" "SYSTEM MESSAGES"("Versão 1.0.25 (//2025)  - Reformulação controle da trapeira. Sensor da plataforma. Alarmes meteorológicos. Bridge serial." ("message")) -> ()
    }
  }
  n177 = while "MAIN - While Loop" {
    tunnel: ["sair"] -> w1
    stop <- w92 stop-if-true
    # "100"
    # "Não Alterar esse Parametro"
    n178 = stacked-sequence "PRINCIPAL - Stacked Sequence Structure" {
      seq-local: [w97 _ _ _ _ _] -> [_ w100 _ _ _ w4164]
      frame #0 {
        # "CLIENTE REMOTO"
        # "Verifica se Existe Cliente Remoto Conectado"
        n179 = invoke class="VI" method="RP.Client Connections"() -> ("Connections"=w98:T10, "Controller"=w96:i32)  [unwired: 5 in, 3 out]
        n180 = Tick Count (ms)() -> (millisecond timer value=w97:u32)
        n181 = Equal?(x=w96, y=0) -> (x = y?=→"Remote User in Control":bool)
        n182 = global write "Global_Telescopio.vi" "Controller Rem/Loc"(w96) -> ()
        n183 = global write "Global_Telescopio.vi" "Dados do Computador Remoto Conectado"(w98) -> ()
      }
      frame #1 {
        # "ACOES CONTINUAS"
        n184 = stacked-sequence "MONITORACAO - Stacked Sequence Structure" {
          tunnel: w100 -> [_ _ _ w475 _ _ _ _ _ _ _ _ _ _ _ _]
          frame #0 {
            w122 = u16 3 items=["ZERO", "AH", "DEC", "TUBO", "CUP", "CASS", "COUDE"] ("Controlador")
            w130 = u16 4 items=["ZERO", "AH", "DEC", "TUBO", "CUP", "CASS", "COUDE"] ("Controlador")
            w131 = u16 2 items=["ZERO", "AH", "DEC", "TUBO", "CUP", "CASS", "COUDE"] ("Controlador")
            w134 = u16 1 items=["ZERO", "AH", "DEC", "TUBO", "CUP", "CASS", "COUDE"] ("Controlador")
            # "PROCESSO LE ENCODERS"
            # "LEITURA STATUS DOS CONTROLADORES"
            n185 = flat-sequence {
              tunnel: ["Case Constant\n(See Context Help)"] -> w114
              frame #0 {
                n186 = Tick Count (ms)() -> (millisecond timer value=w137:u32)
                n187 = global write "Global_Telescopio.vi" "ExecTime"(w137) -> ()
              }
            }
            n188 = disable-structure shown="Enabled" {
              frame Disabled {
                # "TU safe"
                # "ZeroMQ"
                # "Grava o valor do foco \natual a cada minuto"
                n189 = call "Get host time.vi"() -> ("BR current time"=w158:timestamp)  [unwired: 8 in, 3 out]
                n190 = Format Date/Time String(time format string (%c)="%S", seconds (now)=w158) -> (date/time string=w161:string)  [unwired: 1 in]
                n191 = Equal?(x=w161, y="00") -> (x = y?=w159:bool)
                n192 = case shown="True" w159 {
                  frame False {
                  }
                  frame True {
                    n193 = local read "Foco"() -> (w165:dbl)
                    n194 = Number To Decimal String(number=w165) -> (decimal integer string=w164:string)  [unwired: 1 in]
                    n195 = call "Log_Foco.vi"("command"=" ", "focValue"=w164, "pathLogFocoString"="C:\\TCS\\LOG\\FOCO\\") -> ()  [unwired: 6 in]
                  }
                }
              }
              frame Enabled {
                # "ZeroMQ"
                n196 = First Call?() -> (First Call?: T/F=w167:bool)
                n197 = case shown="True" w167 {
                  frame False {
                  }
                  frame True {
                    n198 = global read "Global_Telescopio.vi" "transactionId0MQ"() -> (w168:u64)
                    n199 = Increment(x=w168) -> (x+1=w169:u64)
                    n200 = call "Focus PUSH.vi"("action"="STATUS" ("controller"), "clientTransactionId"=w168) -> ()  [unwired: 9 in, 1 out]
                    n201 = global write "Global_Telescopio.vi" "transactionId0MQ"(w169) -> ()
                  }
                }
              }
            }
            n202 = case shown="False" w114 {
              selector: w114 -> [_ w233]
              tunnel: [w232 w233] -> w132
              tunnel: w131 -> [w231 _]
              tunnel: [w230 _] -> w133
              tunnel: [w229 _] -> w105
              tunnel: [w228 _] -> w118
              frame False {
                n203 = call "Get Status Controlador.vi"("Controlador"=w231) -> ("Status"=w228:string, "Parametros"=w230:string, "Bits Status"=w229:bool[], "Erro comunicação"=w232:bool)
              }
              frame True {
              }
            }
            "DEC_STAT" <- w118
            "DEC" <- w105
            n204 = case shown="False" w114 {
              selector: w114 -> [_ w227]
              tunnel: [w226 w227] -> w129
              tunnel: w130 -> [w225 _]
              tunnel: [w224 _] -> w128
              tunnel: [w223 _] -> w115
              tunnel: [w222 _] -> w117
              frame False {
                n205 = call "Get Status Controlador.vi"("Controlador"=w225) -> ("Status"=w222:string, "Parametros"=w224:string, "Bits Status"=w223:bool[], "Erro comunicação"=w226:bool)
              }
              frame True {
              }
            }
            "CUP_STAT" <- w117
            "CUP" <- w115
            n206 = case shown="False" w114 {
              selector: w114 -> [_ w189]
              tunnel: [w188 w189] -> w123
              tunnel: w122 -> [w187 _]
              tunnel: [w186 _] -> w124
              tunnel: [w185 _] -> w113
              tunnel: [w184 _] -> w116
              frame False {
                n207 = call "Get Status Controlador.vi"("Controlador"=w187) -> ("Status"=w184:string, "Parametros"=w186:string, "Bits Status"=w185:bool[], "Erro comunicação"=w188:bool)
              }
              frame True {
              }
            }
            "TUBO_STAT" <- w116
            "TUBO" <- w113
            n208 = case shown="False" w114 {
              selector: w114 -> [_ w267]
              tunnel: w134 -> [w266 _]
              tunnel: [w265 _] -> w106
              tunnel: [w264 _] -> w136
              tunnel: [w263 w267] -> w135
              tunnel: [w262 _] -> w119
              frame False {
                n209 = call "Get Status Controlador.vi"("Controlador"=w266) -> ("Status"=w262:string, "Parametros"=w264:string, "Bits Status"=w265:bool[], "Erro comunicação"=w263:bool)
              }
              frame True {
              }
            }
            "AH_STAT" <- w119
            "RA" <- w106
            n210 = call "Testa_Comunicação.vi"("DEC"=w105, "RA"=w106) -> ()  [unwired: 10 in]
            n211 = Index Array(array=w113, index=3) -> (element=w111:bool)
            n212 = case shown="False" w111 {
              tunnel: ["S" "M"] -> w110
              frame False {
              }
              frame True {
              }
            }
            n213 = case shown="False" w135 {
              tunnel: w106 -> [w254 _]
              tunnel: w136 -> [w253 _]
              tunnel: [w251 _] -> w121
              frame False {
                # "Leitura Válida"
                n214 = call <vilib>:"Trim Whitespace.vi"("string"=w253) -> ("trimmed string"=w251:string)  [unwired: 1 in]
                n215 = call "hms_rad.vi"("True = hora"=TRUE, "Texto Graus"=w251) -> ("radianos"=w248:dbl)  [unwired: 3 in]
                n216 = global write "Global_Telescopio.vi" "StatusAH"(w254) -> ()
                n217 = global read "Global_Telescopio.vi" "PosAH"() -> (w250:dbl)
                n218 = Equal?(x=w250, y=w248) -> (x = y?=w249:bool)
                n219 = case shown="False" w249 {
                  tunnel: w248 -> [w257 _]
                  frame False {
                    w256 = 0 ("CR AH")
                    n220 = global write "Global_Telescopio.vi" "PosAH"(w257) -> ()
                    n221 = local write "CR AH"(w256) -> ()
                    n222 = local write "CR AH UTILS"(w256) -> ()
                    "PosAH" <- w257
                    "Flag ativo AH" <- TRUE ("Flag ativo AH")
                  }
                  frame True {
                    n223 = local read "CR AH UTILS"() -> (w259:i32)
                    n224 = local read "CR AH"() -> (w260:i32)
                    n225 = Increment(x=w259) -> (x+1=w258:i32)
                    n226 = Increment(x=w260) -> (x+1=w261:i32)
                    n227 = local write "CR AH UTILS"(w258) -> ()
                    n228 = local write "CR AH"(w261) -> ()
                  }
                }
              }
              frame True {
                # "Erro na Leitura"
              }
            }
            "AH_ENC" <- w121
            n229 = case shown="False" w132 {
              tunnel: w133 -> [w239 _]
              tunnel: w105 -> [w238 _]
              tunnel: [w237 _] -> w120
              frame False {
                # "Leitura Válida"
                n230 = call <vilib>:"Trim Whitespace.vi"("string"=w239) -> ("trimmed string"=w237:string)  [unwired: 1 in]
                n231 = global write "Global_Telescopio.vi" "StatusDEC"(w238) -> ()
                n232 = call "hms_rad.vi"("True = hora"=FALSE, "Texto Graus"=w237) -> ("radianos"=w234:dbl)  [unwired: 3 in]
                n233 = global read "Global_Telescopio.vi" "PosDEC"() -> (w236:dbl)
                n234 = Equal?(x=w236, y=w234) -> (x = y?=w235:bool)
                n235 = case shown="False" w235 {
                  tunnel: w234 -> [w243 _]
                  frame False {
                    w242 = 0 ("CR DEC")
                    n236 = global write "Global_Telescopio.vi" "PosDEC"(w243) -> ()
                    n237 = local write "CR DEC UTILS"(w242) -> ()
                    n238 = local write "CR DEC"(w242) -> ()
                    "PosDEC" <- w243
                    "Flag ativo DEC" <- TRUE ("Flag ativo DEC")
                  }
                  frame True {
                    n239 = local read "CR DEC UTILS"() -> (w245:i32)
                    n240 = local read "CR DEC"() -> (w247:i32)
                    n241 = Increment(x=w245) -> (x+1=w244:i32)
                    n242 = Increment(x=w247) -> (x+1=w246:i32)
                    n243 = local write "CR DEC UTILS"(w244) -> ()
                    n244 = local write "CR DEC"(w246) -> ()
                  }
                }
              }
              frame True {
                # "Erro na Leitura"
              }
            }
            "DEC_ENC" <- w120
            n245 = case shown="False" w129 {
              tunnel: w115 -> [w197 _]
              tunnel: w128 -> [w196 _]
              tunnel: [w195 w220] -> w103
              tunnel: [w194 w221] -> w104
              tunnel: [w192 FALSE] -> w102
              frame False {
                w193 = u16 12 items=["Alarme", "Atencao", "Erro", "Ocupado", "TBD", "LCB", "Trapeira", "Paravento", "DomoRap", "DomoCW", "DomoCCW", "TBD", "Em movimento", "TBD"] ("NomeStatus")
                # "Leitura Válida"
                n246 = global write "Global_Telescopio.vi" "StatusCUP"(w197) -> ()
                n247 = stacked-sequence {
                  tunnel: w196 -> [w203 _ _]
                  tunnel: [w199 _ _] -> w195
                  tunnel: [_ w208 _] -> w194
                  tunnel: [_ _ w210] -> w190
                  tunnel: w193 -> [_ _ w215]
                  tunnel: [w198 _ _] -> w191
                  frame #0 {
                    n248 = call <vilib>:"Trim Whitespace.vi"("string"=w203) -> ("trimmed string"=w199:string)  [unwired: 1 in]
                    n249 = Decimal String To Number(string=w199) -> (number=w202:i32)  [unwired: 2 in, 1 out]
                    n250 = global read "Global_Telescopio.vi" "CupLastEnc"() -> (w201:string)
                    n251 = global write "Global_Telescopio.vi" "PosCUP"(w202) -> ()
                    n252 = Not Equal?(x=w199, y=w201) -> (x != y?=w200:bool)
                    n253 = case shown="True" w200 {
                      tunnel: w199 -> [_ w207]
                      tunnel: [TRUE FALSE] -> w198
                      frame False {
                      }
                      frame True {
                        n254 = call "TickTimeout.vi"() -> ("msTick"=w206:u32)  [unwired: 2 in, 2 out]
                        n255 = global write "Global_Telescopio.vi" "CupLastEnc"(w207) -> ()
                        n256 = global write "Global_Telescopio.vi" "CupTimeLock"(w206) -> ()
                      }
                    }
                  }
                  frame #1 {
                    n257 = global read "Global_Telescopio.vi" "PosCUP"() -> (w209:i16)
                    n258 = call "Checa destino cupula.vi"("Target"=w209) -> ("angCUP"=w208:string)  [unwired: 6 in, 2 out]
                  }
                  frame #2 {
                    n259 = global read "Global_Telescopio.vi" "CupTimeLock"() -> (w214:u32)
                    n260 = call "Bit Status CUP.vi"("NomeStatus"=w215) -> ("StatBit"=w211:bool)
                    n261 = call "TickTimeout.vi"("msInicial"=w214, "msTimeout"=u32 10000) -> ("Timeout"=w212:bool)  [unwired: 2 out]
                    n262 = Select(t=u32 16747264 ("orangeColor"), s=w211, f=u32 16776376 ("yellowColor")) -> (s? t:f=w218:u32)
                    n263 = And(x=w212, y=w211) -> (x .and. y?=w210:bool)
                    n264 = property on="angCup" class="Str"("Text.BGColor"=w218) -> ()  [unwired: 2 in, 2 out]
                  }
                }
                n265 = And(x=w190, y=w191) -> (x .and. y?=w192:bool)
              }
              frame True {
                # "Erro na Leitura"
                n266 = local read "DOMO_ENC"() -> (w220:string)
                n267 = local read "angCup"() -> (w221:string)
              }
            }
            "DOMO_ENC" <- w103
            "angCup" <- w104
            n268 = global write "Global_Telescopio.vi" "MOTOR LIGADO"(w110) -> ()
            n269 = case shown="False" w123 {
              tunnel: w113 -> [w182 _]
              tunnel: w124 -> [w177 _]
              frame False {
                # "Leitura Válida"
                n270 = call <vilib>:"Trim Whitespace.vi"("string"=w177) -> ("trimmed string"=w181:string)  [unwired: 1 in]
                n271 = Decimal String To Number(string=w181) -> (number=w180:i32)  [unwired: 2 in, 1 out]
                n272 = global write "Global_Telescopio.vi" "StatusTUBO"(w182) -> ()
                n273 = global write "Global_Telescopio.vi" "PosFOCO"(w180) -> ()
                n274 = String Subset(string=w177, offset (0)=10, length (rest)=1 ("length (rest)")) -> (substring=→"EspAtual":string)
                n275 = Number To Decimal String(number=w180) -> (decimal integer string=w175:string)  [unwired: 1 in]
                "FOCO_ENC" <- w175
                n276 = Decimal String To Number(string=w175) -> (number=w173:i32)  [unwired: 2 in, 1 out]
                n277 = Greater Than 0?(x=w173) -> (x > 0?=w174:bool)
                n278 = case shown="True" w174 {
                  tunnel: w173 -> [_ w183]
                  frame False {
                  }
                  frame True {
                    n279 = global write "Global_Telescopio.vi" "Foco"(w183) -> ()
                  }
                }
              }
              frame True {
                # "Erro na Leitura"
              }
            }
            n280 = local read "LedPointing"() -> (w108:bool)
            n281 = local read "MOVING"() -> (w109:bool)
            n282 = case shown="True" w102 {
              tunnel: w103 -> [_ w151]
              frame False {
              }
              frame True {
                w152 = "\t"
                # "TU safe"
                # "CÚPULA TRAVADA: Write LOG"
                n283 = String To Path(string="C:\\TCS\\LOG\\CUPULA\\TRAVOU.TXT" ("pathLogFocoString")) -> (path=w157:path)
                n284 = Open/Create/Replace File(file path (use dialog)=w157, error in=errorcluster {"status"=FALSE, "code"=0, "source"=""}, operation (0:open)=T7."open or create") -> (refnum out=w147:refnum<file>, error out=w145:errorcluster)  [unwired: 3 in, 1 out]
                n285 = call "Safe Date-Time String.vi"() -> ("Safe time string"=w139:string, "Safe date string"=w140:string)  [unwired: 3 in]
                n286 = Build Array(w140, w152, w139, w152, "ETIQUETA: ", w151, "\r\n") -> (w148:string[])
                n287 = call "TickTimeout.vi"() -> ("msTick"=w141:u32)  [unwired: 2 in, 2 out]
                n288 = Set File Position(refnum=w147, from (0:start)=enum16{"start", "end", "current"}."end", error in=w145) -> (refnum out=w146:refnum<file>, error out=w144:errorcluster)  [unwired: 1 in]
                n289 = global write "Global_Telescopio.vi" "CupTimeLock"(w141) -> ()
                n290 = Write to Text File(file (use dialog)=w146, text=w148, error in=w144) -> (refnum out=w154:refnum<file>, error out=w155:errorcluster)  [unwired: 1 in, 1 out]
                n291 = Close File(refnum=w154, error in=w155) -> ()  [unwired: 2 out]
              }
            }
            n292 = Or(x=w108, y=w109) -> (x .or. y?=w107:bool)
            n293 = shared-variable "My Computer\\Shared_160.lvlib\\Beep"(w107) -> ()  [unwired: 1 in, 1 out]
            n294 = call "Sideral_Time.vi"("Fuso"=-3.0) -> ("TU"=→"UT":string, "Sideral Time"=w125:dbl)  [unwired: 2 in, 1 out]
            n295 = global write "Global_Telescopio.vi" "Sideral Time"(w125) -> ()
          }
          frame #1 {
            w286 = u16 9 items=["Alarme", "Atencao", "Erro", "Ocupado", "Protecao", "Embreagem", "Tracking", "Var. Track", "Rápido", "Ligeiro", "Médio", "Lento", "Em movimento", ""] ("NomeStatus")
            w287 = u16 9 items=["Alarme", "Atencao", "Erro", "Ocupado", "Protecao", "Embreagem", "Tracking", "Var. Track", "Rápido", "Ligeiro", "Médio", "Lento", "Em movimento", ""] ("NomeStatus")
            w290 = u16 8 items=["Alarme", "Atencao", "Erro", "Ocupado", "Protecao", "Embreagem", "Tracking", "Var. Track", "Rápido", "Ligeiro", "Médio", "Lento", "Em movimento", ""] ("NomeStatus")
            w291 = u16 8 items=["Alarme", "Atencao", "Erro", "Ocupado", "Protecao", "Embreagem", "Tracking", "Var. Track", "Rápido", "Ligeiro", "Médio", "Lento", "Em movimento", ""] ("NomeStatus")
            w297 = 6.283185307179586
            # "20270728"
            # "Desabilita botões \"Precess\" e \"Clear\"\ndurante o apontamento"
            # "MUDANÇA:\nBit EMBREAGEM trocado pelos bits RAPIDO e LIGEIRO para detectar a retirada do objeto da posição centrada."
            # "MUDANÇA FUTURA:\nTrocar globais de calagem por valores \"latch\" dessas globais. Finalidade: manter display de coordenadas consistentes mesmo quando o usuário zerar as calagens, especialmente a local, para o próximo apontamento."
            # "ATUALIZA \nINDICADORES \nDO PAINEL"
            n296 = Tick Count (ms)() -> (millisecond timer value=w269:u32)
            n297 = global read "Global_Telescopio.vi" "ExecTime"() -> (w270:u32)
            n298 = call "Calcula epoch.vi"() -> ("epoch"=→"Epoch":dbl)  [unwired: 2 in]
            n299 = local read "ChkCalGlobal"() -> (w302:bool)
            n300 = global read "Global_Telescopio.vi" "Sideral Time"() -> (w307:dbl)
            n301 = global read "Global_Telescopio.vi" "ObjCentrado"() -> (w271:bool)
            "ObjCentrado" <- w271
            n302 = global read "Global_Telescopio.vi" "PosDEC"() -> (w305:dbl)
            n303 = global read "Global_Telescopio.vi" "PosAH"() -> (w306:dbl)
            n304 = local read "externalNST"() -> (w274:bool)
            n305 = call "Bit Status AH.vi"("NomeStatus"=w291) -> ("StatBit"=w289:bool)
            n306 = call "Bit Status AH.vi"("NomeStatus"=w286) -> ("StatBit"=w285:bool)
            n307 = call "Bit Status DEC.vi"("NomeStatus"=w290) -> ("StatBit"=w283:bool)
            n308 = call "Bit Status DEC.vi"("NomeStatus"=w287) -> ("StatBit"=w284:bool)
            n309 = Subtract(x=w269, y=w270) -> (x-y=→"statusReadTime":u32)
            n310 = local read "LedPointing"() -> (w276:bool)
            n311 = Compound Arithmetic op=OR(w289, w285, w283, w284) -> (w288:bool)
            n312 = case shown="True" w288 {
              frame False {
              }
              frame True {
                n313 = global write "Global_Telescopio.vi" "ObjCentrado"(FALSE) -> ()
              }
            }
